vi "Polynomials Composition.vi"   [LabVIEW 2020, in "NI_AALPro.lvlib"]
doc: "Computes the composition of polynomials <B>P(x)</B> and <B>Q(x)</B>. The data types you wire to the <B>P(x)</B> and <B>Q(x)</B> inputs determine the polymorphic instance to use."
uses:
  <vilib>/Analysis/NI_AALPro.lvlib
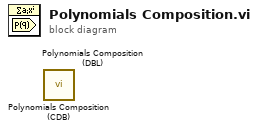
[diagram p0: block diagram]
diagram:
  n1 = call <vilib>:"Polynomials Composition (CDB).vi"() -> ()  [unwired: 10 in, 2 out]
  n2 = call <vilib>:"Polynomials Composition (DBL).vi"() -> ()  [unwired: 10 in, 2 out]
